vi "Read position(x,y).vi"(8 "error in (no error)":errorcluster, 11 "Object in":refnum<class "Object.lvclass">) -> (0 "error out":errorcluster, 2 "position(x,y)":dbl[](array[numeric]), 3 "Object out":refnum<class "Object.lvclass">)   [LabVIEW 2020, in "Object.lvclass"]
uses:
  Object.lvclass
  Object.lvclass/Object.ctl
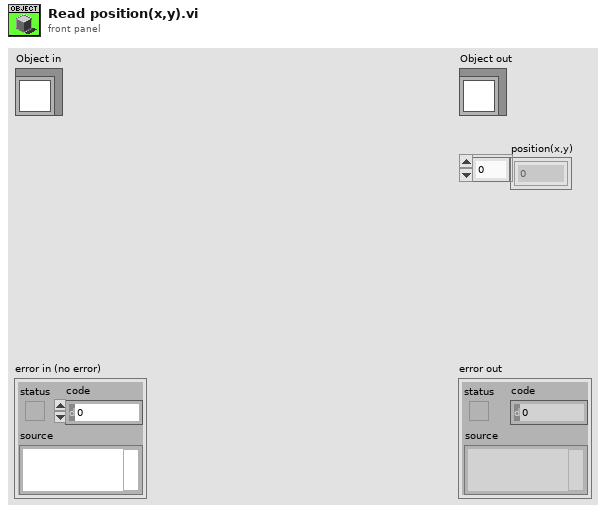
[diagram p1: front panel]
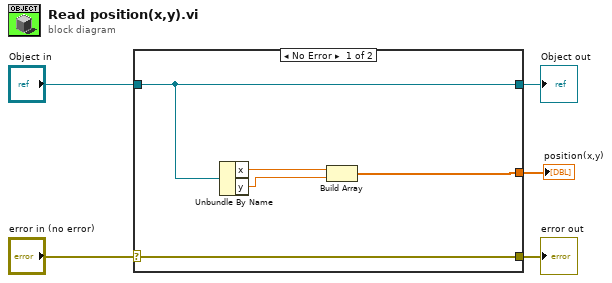
[diagram p0: block diagram]
diagram:
  n1 = case shown="No Error" "error in (no error)" {
    selector: "error in (no error)" -> [w10 w11]
    tunnel: [w10 w11] -> w4
    tunnel: [w9 w12] -> w2
    tunnel: "Object in" -> [w9 w12]
    tunnel: [w6 _] -> w1
    frame No Error {
      n2 = Unbundle By Name(w9) -> ("x"=w8:dbl, "y"=w7:dbl)
      n3 = Build Array(w8, w7) -> (w6:dbl[])
    }
    frame Error {
    }
  }
  "error out" <- w4
  "Object out" <- w2
  "position(x,y)" <- w1
